vi "Set Timestamp Definition.vi"(10 "Timestamp Definition":T1, 11 "Timestamp in":refnum<class "Timestamp.lvclass">) -> (3 "Timestamp out":refnum<class "Timestamp.lvclass">)   [LabVIEW 2020, in "Conditu2.lvlib" / "Columns.lvlib" / "Timestamp.lvclass"]
uses:
  Timestamp.lvclass
  Definition.ctl
  Timestamp.lvclass/Timestamp.ctl
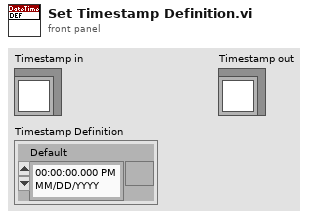
[diagram p1: front panel]
types:
  T1 = typedef "Conditu2.lvlib/Columns.lvlib/Timestamp.lvclass/Definition.ctl" = cluster{"Default":timestamp}
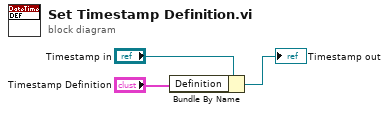
[diagram p0: block diagram]
diagram:
  n1 = Bundle By Name(cluster="Timestamp in", "Definition"="Timestamp Definition") -> (→"Timestamp out":refnum<class "Timestamp.lvclass">)
